vi "USB6343_Control_v1.6.5.vi"(8 "error in":errorcluster caption="错误输出", 10 "interface":T2, 11 "tasks":T3) -> ()   [LabVIEW 2013]
uses:
  <vilib>/DAQmx/read.llb/DAQmx Read (Analog 1D DBL NChan 1Samp).vi
  <vilib>/DAQmx/read.llb/DAQmx Read (Digital 1D Bool NChan 1Samp 1Line).vi
  <vilib>/DAQmx/read.llb/DAQmx Read (Counter DBL 1Chan 1Samp).vi
  <vilib>/DAQmx/write.llb/DAQmx Write (Digital 1D Bool NChan 1Samp 1Line).vi
  <vilib>/DAQmx/write.llb/DAQmx Write (Analog 1D DBL NChan 1Samp).vi
  current_position.vi
  <vilib>/DAQmx/miscellaneous.llb/DAQmx Fill In Error Info.vi
  <vilib>/DAQmx/configure/timing.llb/DAQmx Timing (Implicit).vi
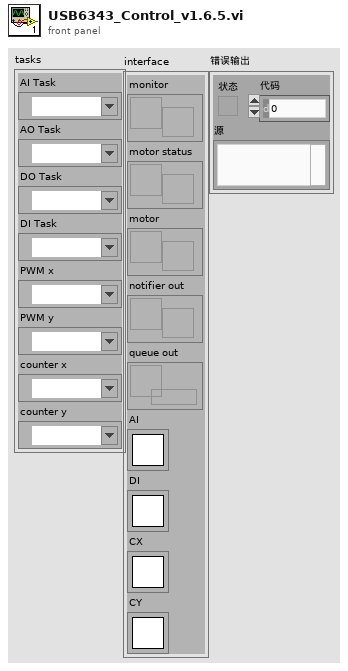
[diagram p1: front panel]
types:
  T1 = typedef "Semaphore RefNum" = refnum<k1>
  T2 = cluster{"monitor":refnum<user-event>, "motor status":refnum<user-event>, "motor":refnum<user-event>, "notifier out":refnum<notifier>, "queue out":refnum<queue>, "AI":T1, "DI":T1, "CX":T1, "CY":T1}
  T3 = cluster{"AI Task":refnum<k21>, "AO Task":refnum<k21>, "DO Task":refnum<k21>, "DI Task":refnum<k21>, "PWM x":refnum<k21>, "PWM y":refnum<k21>, "counter x":refnum<k21>, "counter y":refnum<k21>}
  T4 = cluster{"cmd":string, "channel":i32, "value":dbl, "on/off":bool, "return value":refnum<vi>}
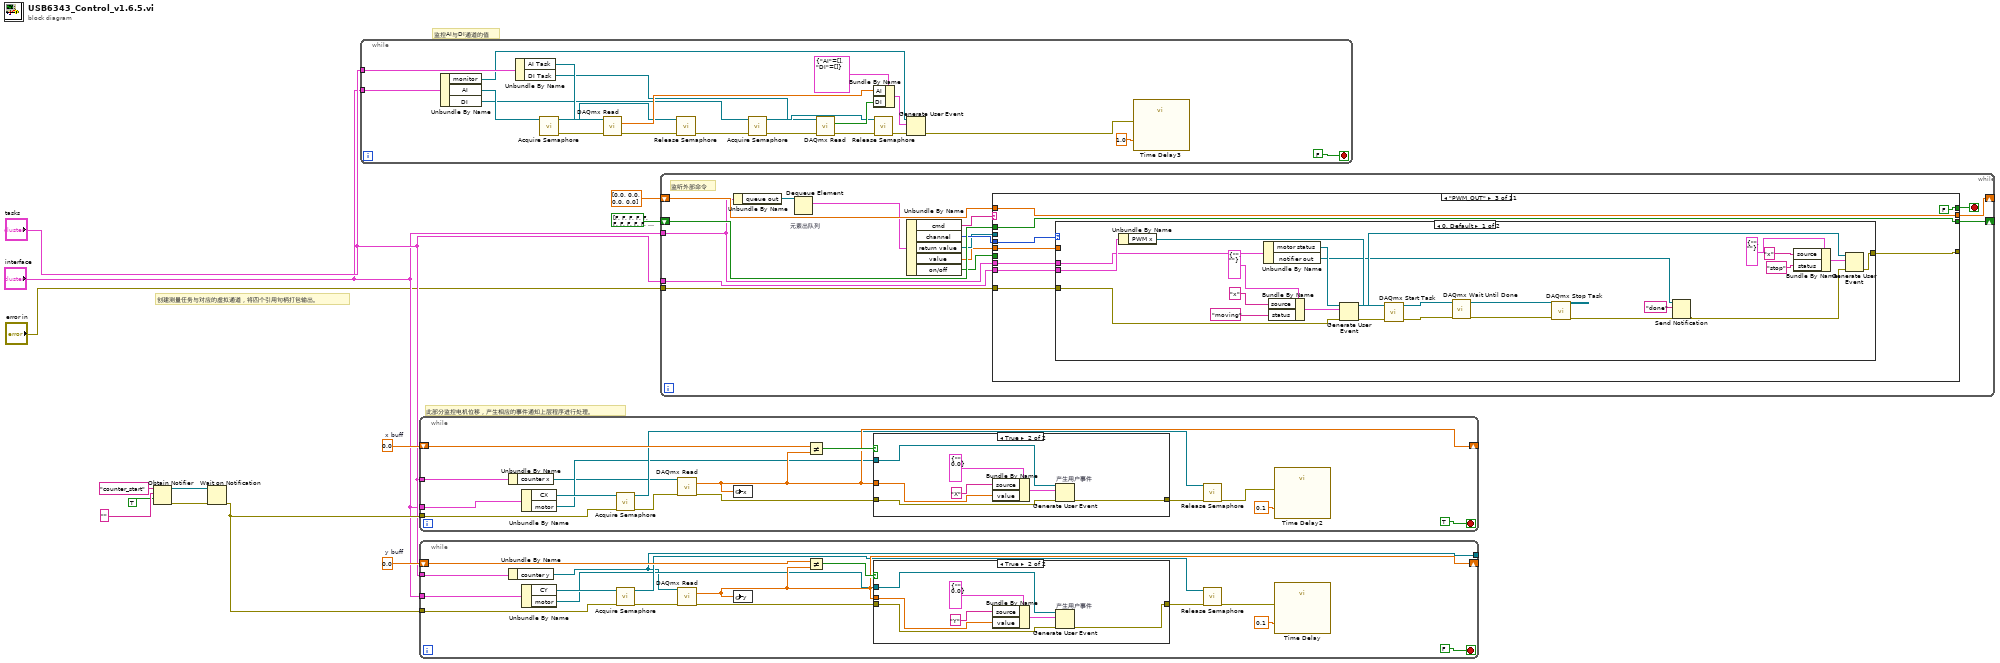
[diagram p0: block diagram]
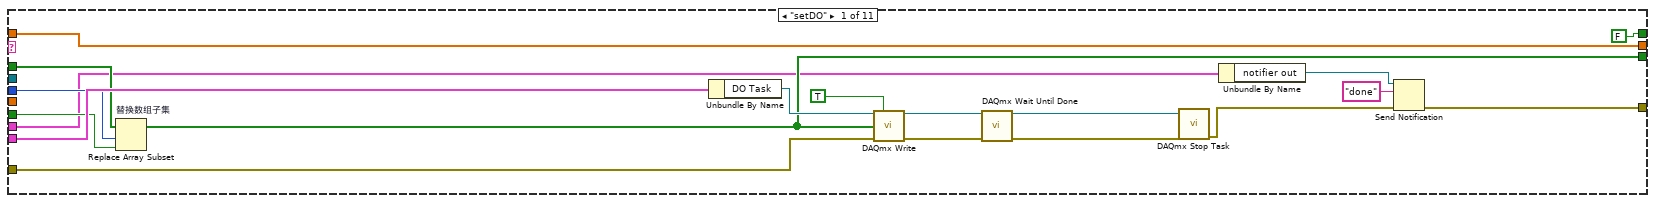
[diagram p4: hidden frame]
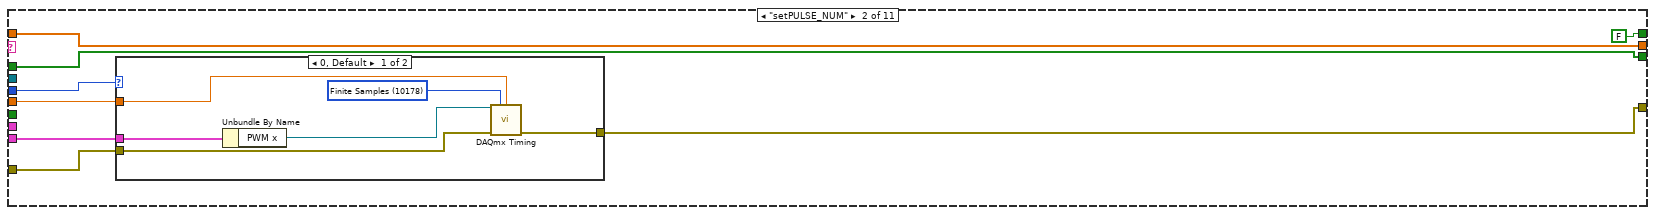
[diagram p5: hidden frame]
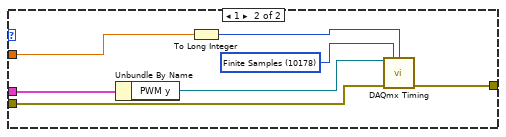
[diagram p6: hidden frame]
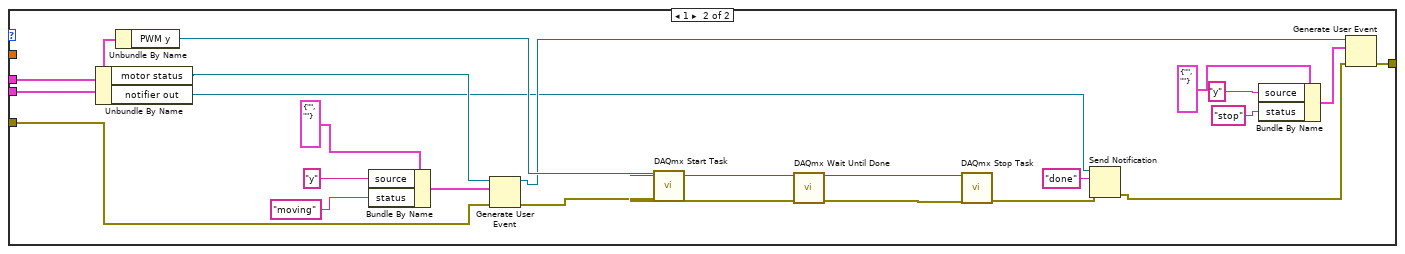
[diagram p7: hidden frame]
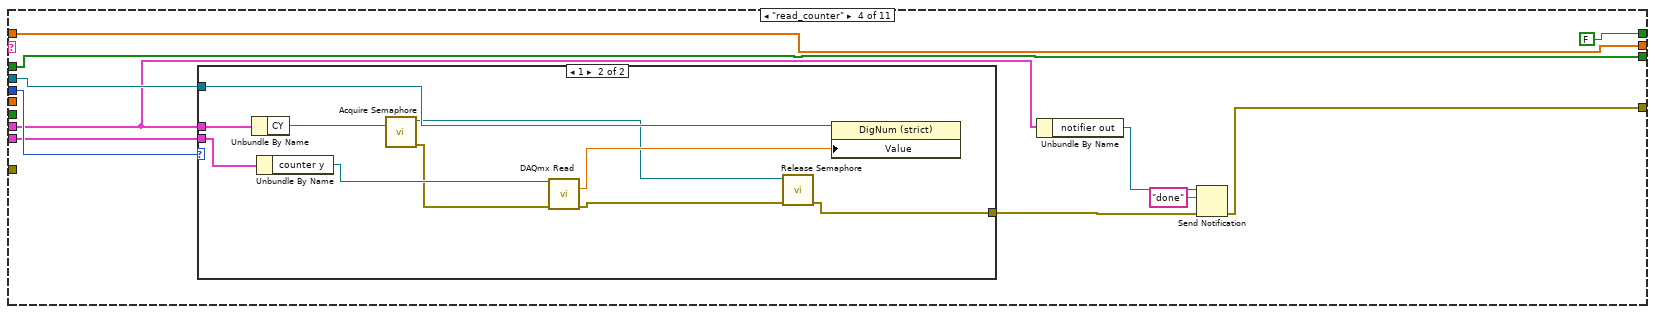
[diagram p8: hidden frame]
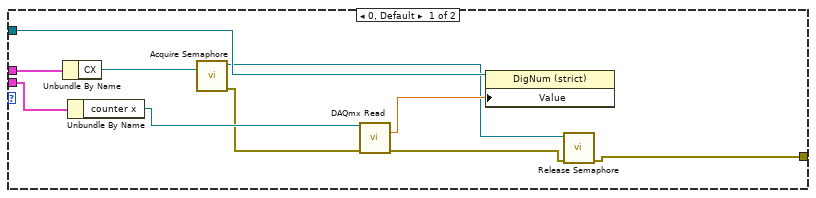
[diagram p9: hidden frame]
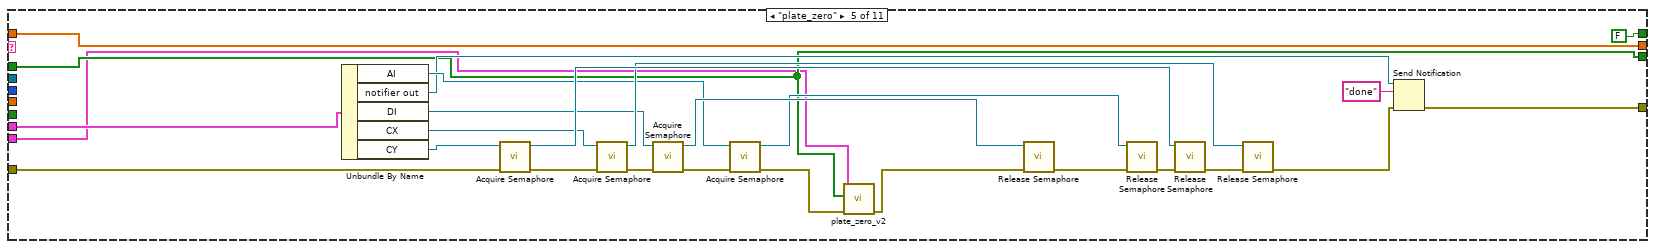
[diagram p10: hidden frame]
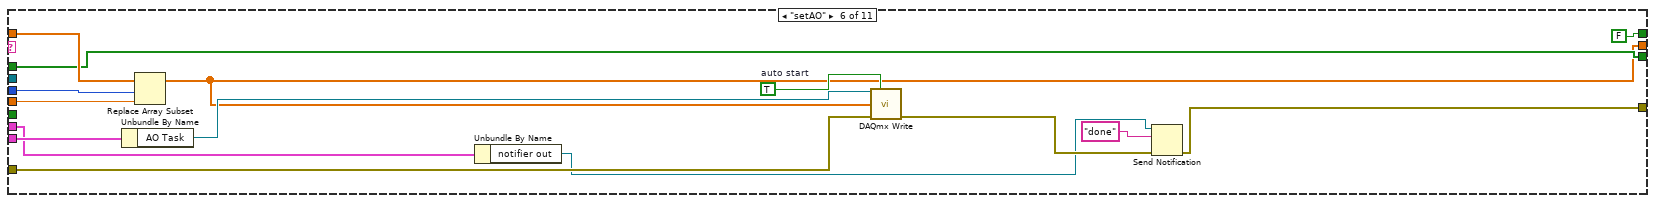
[diagram p11: hidden frame]
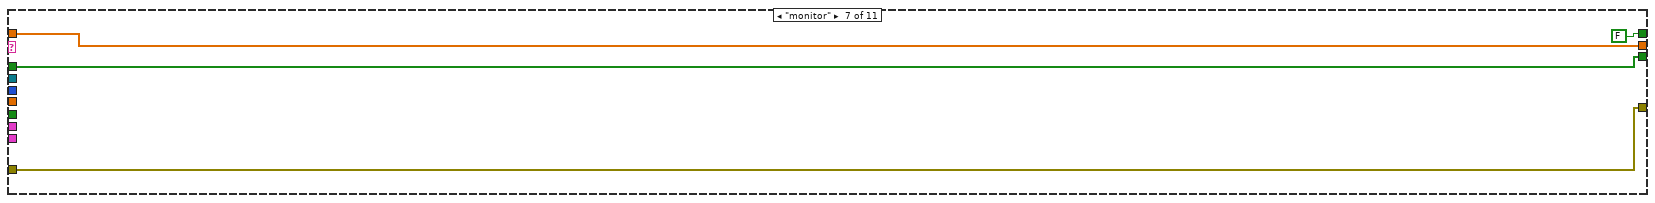
[diagram p12: hidden frame]
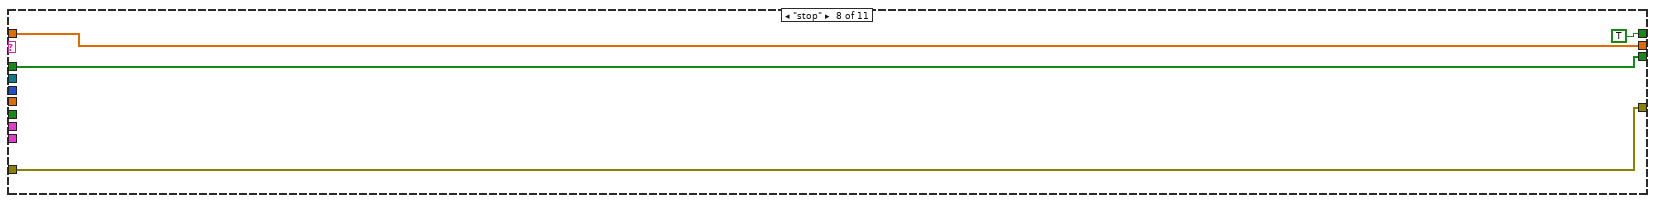
[diagram p13: hidden frame]
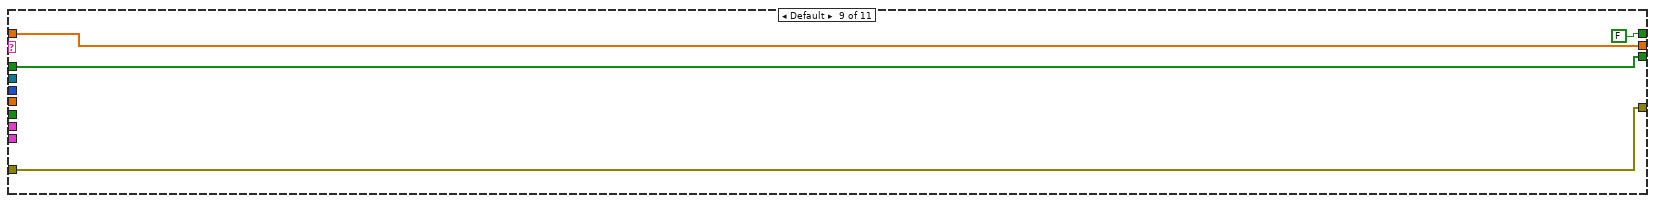
[diagram p14: hidden frame]
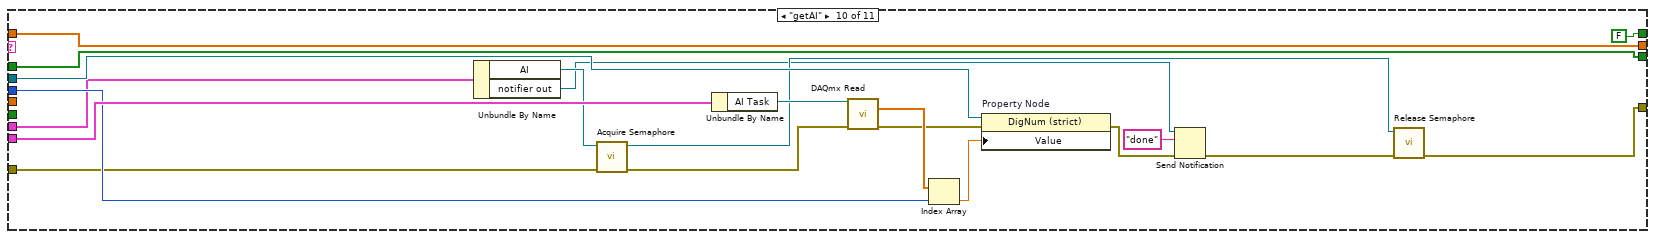
[diagram p15: hidden frame]
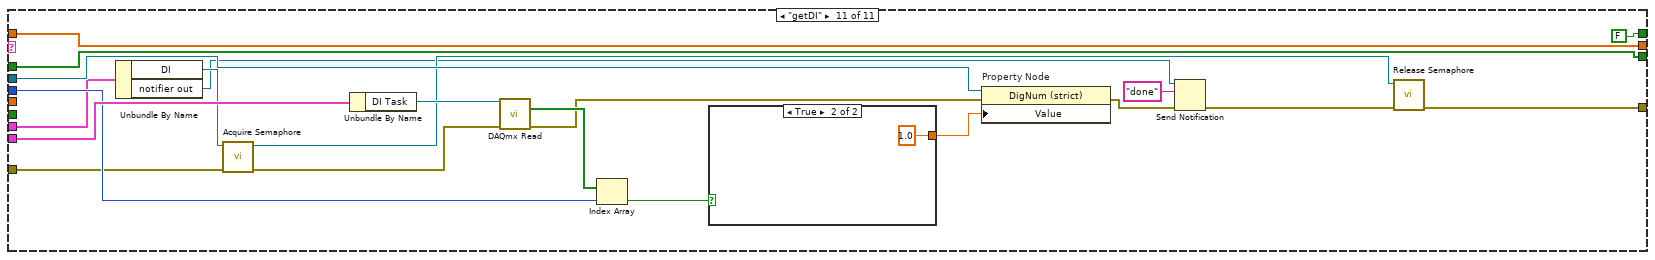
[diagram p16: hidden frame]
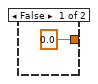
[diagram p17: hidden frame]
diagram:
  w10 = 0.0  # x buff
  w11 = 0.0  # y buff
  # "监控AI与DI通道的值"
  # "此部分监控电机位移，产生相应的事件通知上层程序进行处理。"
  # "创建测量任务与对应的虚拟通道，将四个引用句柄打包输出。"
  n1 = Obtain Notifier(name (unnamed)="counter_start", notification data type="", create if not found? (T)=TRUE) -> (notifier out=w6:refnum<notifier>, error out=w7:errorcluster)  [unwired: 1 in, 1 out]
  n2 = Wait on Notification(notifier=w6, error in (no error)=w7) -> (error out=w5:errorcluster)  [unwired: 2 in, 3 out]
  n3 = while {
    tunnel: "tasks" -> [w33]
    tunnel: "interface" -> [w18]
    stop <- FALSE stop-if-true
    n4 = Unbundle By Name(w18) -> ("monitor"=w17:refnum<user-event>, "AI"=w16:T1, "DI"=w15:T1)
    n5 = Unbundle By Name(w33) -> ("AI Task"=w34:refnum<k21>, "DI Task"=w14:refnum<k21>)
    n6 = call <vilib>:"Acquire Semaphore.vi"("semaphore"=w16) -> ("error out"=w19:errorcluster, "semaphore out"=w21:T1)  [unwired: 4 in, 1 out]
    n7 = call-poly <vilib>:"DAQmx Read.vi"("task/channels in"=w34, "error in"=w19) -> ("data"=w31:dbl[], "error out"=w26:errorcluster)  [unwired: 11 in, 1 out]
    n8 = call <vilib>:"Release Semaphore.vi"("error in (no error)"=w26, "semaphore"=w21) -> ("error out"=w25:errorcluster)  [unwired: 4 in, 1 out]
    n9 = call <vilib>:"Acquire Semaphore.vi"("error in (no error)"=w25, "semaphore"=w15) -> ("error out"=w24:errorcluster, "semaphore out"=w20:T1)  [unwired: 3 in, 1 out]
    n10 = call-poly <vilib>:"DAQmx Read.vi"("task/channels in"=w14, "error in"=w24) -> ("data"=w30:bool[], "error out"=w23:errorcluster)  [unwired: 11 in, 1 out]
    n11 = Bundle By Name(cluster=cluster{"AI":dbl[], "DI":bool[]} {"AI"=[], "DI"=[]} ("event data"), "AI"=w31, "DI"=w30) -> (w27:cluster{"AI":dbl[], "DI":bool[]})
    n12 = call <vilib>:"Release Semaphore.vi"("error in (no error)"=w23, "semaphore"=w20) -> ("error out"=w22:errorcluster)  [unwired: 4 in, 1 out]
    n13 = Generate User Event(user event=w17, event data cluster=w27, error in=w22) -> (error out=w29:errorcluster)  [unwired: 1 in, 1 out]
    n14 = call "Time Delay3"("error in (no error)"=w29, "Delay Time (s)"=1.0) -> ()  [unwired: 9 in, 1 out]
  }
  n15 = while {
    shift-right: [w47] -> _
    shift-left: w10 -> [w51]
    tunnel: "interface" -> [w41]
    tunnel: "tasks" -> [w38]
    tunnel: w5 -> [w36]
    stop <- TRUE stop-if-true
    n16 = Unbundle By Name(w38) -> ("counter x"=w37:refnum<k21>)
    n17 = Unbundle By Name(w41) -> ("CX"=w40:T1, "motor"=w39:refnum<user-event>)
    n18 = call <vilib>:"Acquire Semaphore.vi"("error in (no error)"=w36, "semaphore"=w40) -> ("error out"=w46:errorcluster, "semaphore out"=w43:T1)  [unwired: 3 in, 1 out]
    n19 = call-poly <vilib>:"DAQmx Read.vi"("task/channels in"=w37, "error in"=w46) -> ("data"=w47:dbl, "error out"=w49:errorcluster)  [unwired: 11 in, 1 out]
    n20 = global write "current_position.vi" "x"(w47) -> ()
    n21 = Not Equal?(x=w51, y=w47) -> (x != y?=w50:bool)
    n22 = case shown="True" w50 {
      tunnel: w47 -> [_ w53]
      tunnel: w49 -> [w52 w56]
      tunnel: [w52 w55] -> w45
      tunnel: w39 -> [_ w54]
      frame False {
      }
      frame True {
        n23 = Bundle By Name(cluster=cluster{"source":string, "value":dbl} {"source"="", "value"=0.0} ("事件数据"), "source"="X", "value"=w53) -> (w57:cluster{"source":string, "value":dbl})
        n24 = Generate User Event "产生用户事件"(user event=w54, event data cluster=w57, error in=w56) -> (error out=w55:errorcluster)  [unwired: 1 in, 1 out]
      }
    }
    n25 = call <vilib>:"Release Semaphore.vi"("error in (no error)"=w45, "semaphore"=w43) -> ("error out"=w44:errorcluster)  [unwired: 4 in, 1 out]
    n26 = call "Time Delay2"("error in (no error)"=w44, "Delay Time (s)"=0.1) -> ()  [unwired: 9 in, 1 out]
  }
  n27 = while {
    tunnel: [w61] -> _
    shift-right: [w71] -> _
    shift-left: w11 -> [w75]
    tunnel: "interface" -> [w65]
    tunnel: "tasks" -> [w62]
    tunnel: w5 -> [w60]
    stop <- FALSE stop-if-true
    n28 = Unbundle By Name(w62) -> ("counter y"=w61:refnum<k21>)
    n29 = Unbundle By Name(w65) -> ("CY"=w64:T1, "motor"=w63:refnum<user-event>)
    n30 = call <vilib>:"Acquire Semaphore.vi"("error in (no error)"=w60, "semaphore"=w64) -> ("error out"=w70:errorcluster, "semaphore out"=w67:T1)  [unwired: 3 in, 1 out]
    n31 = call-poly <vilib>:"DAQmx Read.vi"("task/channels in"=w61, "error in"=w70) -> ("data"=w71:dbl, "error out"=w73:errorcluster)  [unwired: 11 in, 1 out]
    n32 = global write "current_position.vi" "y"(w71) -> ()
    n33 = Not Equal?(x=w75, y=w71) -> (x != y?=w74:bool)
    n34 = case shown="True" w74 {
      tunnel: w71 -> [_ w77]
      tunnel: w73 -> [w76 w79]
      tunnel: [w76 w78] -> w69
      tunnel: w63 -> [_ w80]
      frame False {
      }
      frame True {
        n35 = Bundle By Name(cluster=cluster{"source":string, "value":dbl} {"source"="", "value"=0.0} ("事件数据"), "source"="Y", "value"=w77) -> (w81:cluster{"source":string, "value":dbl})
        n36 = Generate User Event "产生用户事件"(user event=w80, event data cluster=w81, error in=w79) -> (error out=w78:errorcluster)  [unwired: 1 in, 1 out]
      }
    }
    n37 = call <vilib>:"Release Semaphore.vi"("error in (no error)"=w69, "semaphore"=w67) -> ("error out"=w68:errorcluster)  [unwired: 4 in, 1 out]
    n38 = call "Time Delay"("error in (no error)"=w68, "Delay Time (s)"=0.1) -> ()  [unwired: 9 in, 1 out]
  }
  n39 = while {
    tunnel: "tasks" -> [w92]
    tunnel: "error in" -> [w98]
    shift-right: [w96] -> _
    shift-left: bool[] [FALSE, FALSE, FALSE, FALSE, FALSE, FALSE, FALSE, FALSE, FALSE, FALSE, FALSE, FALSE, FALSE, FALSE, FALSE, FALSE] -> [w97]
    shift-right: [w93] -> _
    shift-left: dbl[] [0.0, 0.0, 0.0, 0.0] ("data") -> [w94]
    tunnel: "interface" -> [w85]
    stop <- w95 stop-if-true
    # "监听外部命令"
    n40 = Unbundle By Name(w85) -> ("queue out"=w84:refnum<queue>)
    n41 = Dequeue Element "元素出队列"(queue=w84) -> (element=w91:T4)  [unwired: 2 in, 3 out]
    n42 = Unbundle By Name(w91) -> ("cmd"=w90:string, "channel"=w89:i32, "return value"=w88:refnum<vi>, "value"=w86:dbl, "on/off"=w87:bool)
    n43 = case shown="\"PWM_OUT\"" w90 {
      tunnel: w89 -> [w115 w119 w141 w206 _ w265 _ _ _ w295 w318]
      tunnel: w92 -> [w117 w122 w144 w205 w228 w267 _ _ _ w299 w320]
      tunnel: w98 -> [w109 w120 w142 _ w244 w260 w268 w272 w276 w288 w308]
      tunnel: w97 -> [w116 w123 w145 w196 w230 w263 w271 w275 w279 w293 w317]
      tunnel: w87 -> [w114 _ _ _ _ _ _ _ _ _ _]
      tunnel: [w107 w123 w145 w196 w230 w263 w271 w275 w279 w293 w317] -> w96
      tunnel: [FALSE FALSE FALSE FALSE FALSE FALSE FALSE TRUE FALSE FALSE FALSE] -> w95
      tunnel: w94 -> [w112 w124 w146 w197 w251 w264 w270 w273 w277 w292 w316]
      tunnel: [w112 w124 w146 w197 w251 w253 w270 w273 w277 w292 w316] -> w93
      tunnel: w88 -> [_ _ _ w204 _ _ _ _ _ w297 w319]
      tunnel: [w111 w118 w140 w199 w250 w257 w268 w272 w276 w284 w303] -> _
      tunnel: w86 -> [_ w121 w143 _ _ w259 _ _ _ _ _]
      tunnel: w85 -> [w103 _ w139 w202 w236 w256 _ _ _ w282 w302]
      frame "setDO" {
        n44 = Replace Array Subset "替换数组子集"(array=w116, new element=w114, index=w115) -> (w107:bool[])
        n45 = Unbundle By Name(w117) -> ("DO Task"=w108:refnum<k21>)
        n46 = call-poly <vilib>:"DAQmx Write.vi"("task/channels in"=w108, "auto start"=TRUE, "data"=w107, "error in"=w109) -> ("task out"=w104:refnum<k21>, "error out"=w105:errorcluster)  [unwired: 9 in, 1 out]
        n47 = call <vilib>:"DAQmx Wait Until Done.vi"("task/channels in"=w104, "error in"=w105) -> ("task out"=w99:refnum<k21>, "error out"=w101:errorcluster)  [unwired: 12 in]
        n48 = call <vilib>:"DAQmx Stop Task.vi"("task/channels in"=w99, "error in"=w101) -> ("error out"=w100:errorcluster)  [unwired: 12 in, 1 out]
        n49 = Unbundle By Name(w103) -> ("notifier out"=w102:refnum<notifier>)
        n50 = Send Notification(notification="done" ("通知"), notifier=w102, error in (no error)=w100) -> (error out=w111:errorcluster)  [unwired: 1 out]
      }
      frame "setPULSE_NUM" {
        n51 = case shown="0, Default" w119 {
          tunnel: w122 -> [w131 w138]
          tunnel: w121 -> [w128 w133]
          tunnel: w120 -> [w127 w135]
          tunnel: [w126 w134] -> w118
          frame 0, Default {
            w129 = 10178 items=["Finite Samples"=10178, "Continuous Samples"=10123, "Hardware Timed Single Point"=12522] ("sample mode")
            n52 = Unbundle By Name(w131) -> ("PWM x"=w130:refnum<k21>)
            n53 = call-poly <vilib>:"DAQmx Timing.vi"("task/channels in"=w130, "sample mode"=w129, "samples per channel"=w128, "error in"=w127) -> ("error out"=w126:errorcluster)  [unwired: 10 in, 1 out]
          }
          frame 1 {
            w136 = 10178 items=["Finite Samples"=10178, "Continuous Samples"=10123, "Hardware Timed Single Point"=12522] ("sample mode")
            n54 = Unbundle By Name(w138) -> ("PWM y"=w137:refnum<k21>)
            n55 = To Long Integer(number=w133) -> (32bit integer=w132:i32)
            n56 = call-poly <vilib>:"DAQmx Timing.vi"("task/channels in"=w137, "sample mode"=w136, "samples per channel"=w132, "error in"=w135) -> ("error out"=w134:errorcluster)  [unwired: 10 in, 1 out]
          }
        }
      }
      frame "PWM_OUT" {
        n57 = case shown="0, Default" w141 {
          tunnel: w144 -> [w171 w195]
          tunnel: w143 -> [_ _]
          tunnel: w142 -> [w163 w187]
          tunnel: [w156 w181] -> w140
          tunnel: w139 -> [w154 w178]
          frame 0, Default {
            n58 = Unbundle By Name(w171) -> ("PWM x"=w170:refnum<k21>)
            n59 = Unbundle By Name(w154) -> ("motor status"=w153:refnum<user-event>, "notifier out"=w148:refnum<notifier>)
            n60 = Bundle By Name(cluster=cluster{"source":string, " status":string} {"source"="", " status"=""} ("event data"), "source"="x", "status"="moving") -> (w161:cluster{"source":string, " status":string})
            n61 = Generate User Event(user event=w153, event data cluster=w161, error in=w163) -> (user event out=w155:refnum<user-event>, error out=w162:errorcluster)  [unwired: 1 in]
            n62 = call <vilib>:"DAQmx Start Task.vi"("task/channels in"=w170, "error in"=w162) -> ("task out"=w168:refnum<k21>, "error out"=w169:errorcluster)  [unwired: 12 in]
            n63 = call <vilib>:"DAQmx Wait Until Done.vi"("task/channels in"=w168, "error in"=w169) -> ("task out"=w167:refnum<k21>, "error out"=w152:errorcluster)  [unwired: 12 in]
            n64 = call <vilib>:"DAQmx Stop Task.vi"("task/channels in"=w167, "error in"=w152) -> ("error out"=w151:errorcluster)  [unwired: 12 in, 1 out]
            n65 = Send Notification(notification="done", notifier=w148, error in (no error)=w151) -> (error out=w150:errorcluster)  [unwired: 1 out]
            n66 = Bundle By Name(cluster=cluster{"source":string, " status":string} {"source"="", " status"=""} ("event data"), "source"="x", "status"="stop") -> (w157:cluster{"source":string, " status":string})
            n67 = Generate User Event(user event=w155, event data cluster=w157, error in=w150) -> (error out=w156:errorcluster)  [unwired: 1 in, 1 out]
          }
          frame 1 {
            n68 = Unbundle By Name(w178) -> ("motor status"=w177:refnum<user-event>, "notifier out"=w172:refnum<notifier>)
            n69 = Unbundle By Name(w195) -> ("PWM y"=w194:refnum<k21>)
            n70 = Bundle By Name(cluster=cluster{"source":string, " status":string} {"source"="", " status"=""} ("event data"), "source"="y", "status"="moving") -> (w180:cluster{"source":string, " status":string})
            n71 = Generate User Event(user event=w177, event data cluster=w180, error in=w187) -> (user event out=w176:refnum<user-event>, error out=w186:errorcluster)  [unwired: 1 in]
            n72 = call <vilib>:"DAQmx Start Task.vi"("task/channels in"=w194, "error in"=w186) -> ("task out"=w192:refnum<k21>, "error out"=w193:errorcluster)  [unwired: 12 in]
            n73 = call <vilib>:"DAQmx Wait Until Done.vi"("task/channels in"=w192, "error in"=w193) -> ("task out"=w190:refnum<k21>, "error out"=w191:errorcluster)  [unwired: 12 in]
            n74 = call <vilib>:"DAQmx Stop Task.vi"("task/channels in"=w190, "error in"=w191) -> ("error out"=w175:errorcluster)  [unwired: 12 in, 1 out]
            n75 = Send Notification(notification="done", notifier=w172, error in (no error)=w175) -> (error out=w174:errorcluster)  [unwired: 1 out]
            n76 = Bundle By Name(cluster=cluster{"source":string, " status":string} {"source"="", " status"=""} ("event data"), "source"="y", "status"="stop") -> (w182:cluster{"source":string, " status":string})
            n77 = Generate User Event(user event=w176, event data cluster=w182, error in=w174) -> (error out=w181:errorcluster)  [unwired: 1 in, 1 out]
          }
        }
      }
      frame "read_counter" {
        n78 = case shown="1" w206 {
          tunnel: w202 -> [w216 w226]
          tunnel: w205 -> [w214 w224]
          tunnel: w204 -> [w211 w221]
          tunnel: [w207 w217] -> w203
          frame 0, Default {
            n79 = Unbundle By Name(w216) -> ("CX"=w215:T1)
            n80 = Unbundle By Name(w214) -> ("counter x"=w213:refnum<k21>)
            n81 = call <vilib>:"Acquire Semaphore.vi"("semaphore"=w215) -> ("error out"=w212:errorcluster, "semaphore out"=w208:T1)  [unwired: 4 in, 1 out]
            n82 = call-poly <vilib>:"DAQmx Read.vi"("task/channels in"=w213, "error in"=w212) -> ("data"=w210:dbl, "error out"=w209:errorcluster)  [unwired: 11 in, 1 out]
            n83 = property class="DigNum (strict)"(reference=w211, "Value"=w210) -> ()  [unwired: 1 in, 2 out]
            n84 = call <vilib>:"Release Semaphore.vi"("error in (no error)"=w209, "semaphore"=w208) -> ("error out"=w207:errorcluster)  [unwired: 4 in, 1 out]
          }
          frame 1 {
            n85 = Unbundle By Name(w226) -> ("CY"=w225:T1)
            n86 = Unbundle By Name(w224) -> ("counter y"=w223:refnum<k21>)
            n87 = call <vilib>:"Acquire Semaphore.vi"("semaphore"=w225) -> ("error out"=w222:errorcluster, "semaphore out"=w218:T1)  [unwired: 4 in, 1 out]
            n88 = call-poly <vilib>:"DAQmx Read.vi"("task/channels in"=w223, "error in"=w222) -> ("data"=w220:dbl, "error out"=w219:errorcluster)  [unwired: 11 in, 1 out]
            n89 = call <vilib>:"Release Semaphore.vi"("error in (no error)"=w219, "semaphore"=w218) -> ("error out"=w217:errorcluster)  [unwired: 4 in, 1 out]
            n90 = property class="DigNum (strict)"(reference=w221, "Value"=w220) -> ()  [unwired: 1 in, 2 out]
          }
        }
        n91 = Unbundle By Name(w202) -> ("notifier out"=w201:refnum<notifier>)
        n92 = Send Notification(notification="done", notifier=w201, error in (no error)=w203) -> (error out=w199:errorcluster)  [unwired: 1 out]
      }
      frame "plate_zero" {
        n93 = Unbundle By Name(w236) -> ("AI"=w235:T1, "notifier out"=w231:refnum<notifier>, "DI"=w234:T1, "CX"=w233:T1, "CY"=w232:T1)
        n94 = call <vilib>:"Acquire Semaphore.vi"("error in (no error)"=w244, "semaphore"=w232) -> ("error out"=w246:errorcluster, "semaphore out"=w240:T1)  [unwired: 3 in, 1 out]
        n95 = call <vilib>:"Acquire Semaphore.vi"("error in (no error)"=w246, "semaphore"=w233) -> ("error out"=w245:errorcluster, "semaphore out"=w237:T1)  [unwired: 3 in, 1 out]
        n96 = call <vilib>:"Acquire Semaphore.vi"("error in (no error)"=w245, "semaphore"=w234) -> ("error out"=w248:errorcluster, "semaphore out"=w239:T1)  [unwired: 3 in, 1 out]
        n97 = call <vilib>:"Acquire Semaphore.vi"("error in (no error)"=w248, "semaphore"=w235) -> ("error out"=w229:errorcluster, "semaphore out"=w238:T1)  [unwired: 3 in, 1 out]
        n98 = call "plate_zero_v2.vi"("error in"=w229, "DO array"=w230, "tasks"=w228) -> ("error out"=w227:errorcluster)  [unwired: 8 in]
        n99 = call <vilib>:"Release Semaphore.vi"("error in (no error)"=w227, "semaphore"=w239) -> ("error out"=w247:errorcluster)  [unwired: 4 in, 1 out]
        n100 = call <vilib>:"Release Semaphore.vi"("error in (no error)"=w247, "semaphore"=w238) -> ("error out"=w243:errorcluster)  [unwired: 4 in, 1 out]
        n101 = call <vilib>:"Release Semaphore.vi"("error in (no error)"=w243, "semaphore"=w240) -> ("error out"=w242:errorcluster)  [unwired: 4 in, 1 out]
        n102 = call <vilib>:"Release Semaphore.vi"("error in (no error)"=w242, "semaphore"=w237) -> ("error out"=w241:errorcluster)  [unwired: 4 in, 1 out]
        n103 = Send Notification(notification="done", notifier=w231, error in (no error)=w241) -> (error out=w250:errorcluster)  [unwired: 1 out]
      }
      frame "setAO" {
        w262 = TRUE  # auto start
        n104 = Unbundle By Name(w267) -> ("AO Task"=w266:refnum<k21>)
        n105 = Replace Array Subset(array=w264, new element=w259, index=w265) -> (w253:dbl[])
        n106 = Unbundle By Name(w256) -> ("notifier out"=w255:refnum<notifier>)
        n107 = call-poly <vilib>:"DAQmx Write.vi"("task/channels in"=w266, "auto start"=w262, "data"=w253, "error in"=w260) -> ("error out"=w258:errorcluster)  [unwired: 9 in, 2 out]
        n108 = Send Notification(notification="done", notifier=w255, error in (no error)=w258) -> (error out=w257:errorcluster)  [unwired: 1 out]
      }
      frame "monitor" {
      }
      frame "stop" {
      }
      frame Default {
      }
      frame "getAI" {
        n109 = Unbundle By Name(w282) -> ("AI"=w281:T1, "notifier out"=w280:refnum<notifier>)
        n110 = call <vilib>:"Acquire Semaphore.vi"("error in (no error)"=w288, "semaphore"=w281) -> ("error out"=w287:errorcluster, "semaphore out"=w283:T1)  [unwired: 3 in, 1 out]
        n111 = Unbundle By Name(w299) -> ("AI Task"=w298:refnum<k21>)
        n112 = call-poly <vilib>:"DAQmx Read.vi"("task/channels in"=w298, "error in"=w287) -> ("data"=w296:dbl[], "error out"=w286:errorcluster)  [unwired: 11 in, 1 out]
        n113 = Index Array(array=w296, index=w295) -> (element=w294:dbl)
        n114 = property on="Property Node" class="DigNum (strict)"(reference=w297, error in=w286, "Value"=w294) -> (error out=w289:errorcluster)  [unwired: 1 out]
        n115 = Send Notification(notification="done" ("通知"), notifier=w280, error in (no error)=w289) -> (error out=w285:errorcluster)  [unwired: 1 out]
        n116 = call <vilib>:"Release Semaphore.vi"("error in (no error)"=w285, "semaphore"=w283) -> ("error out"=w284:errorcluster)  [unwired: 4 in, 1 out]
      }
      frame "getDI" {
        n117 = Unbundle By Name(w302) -> ("DI"=w301:T1, "notifier out"=w300:refnum<notifier>)
        n118 = call <vilib>:"Acquire Semaphore.vi"("error in (no error)"=w308, "semaphore"=w301) -> ("error out"=w307:errorcluster, "semaphore out"=w304:T1)  [unwired: 3 in, 1 out]
        n119 = Unbundle By Name(w320) -> ("DI Task"=w312:refnum<k21>)
        n120 = call-poly <vilib>:"DAQmx Read.vi"("task/channels in"=w312, "error in"=w307) -> ("data"=w311:bool[], "error out"=w306:errorcluster)  [unwired: 11 in, 1 out]
        n121 = Index Array "Index Array"(array=w311, index=w318) -> (element=w310:bool)
        n122 = case shown="True" w310 {
          tunnel: [0.0 1.0] -> w309
          frame False {
          }
          frame True {
          }
        }
        n123 = property on="Property Node" class="DigNum (strict)"(reference=w319, error in=w306, "Value"=w309) -> (error out=w313:errorcluster)  [unwired: 1 out]
        n124 = Send Notification(notification="done" ("通知"), notifier=w300, error in (no error)=w313) -> (error out=w305:errorcluster)  [unwired: 1 out]
        n125 = call <vilib>:"Release Semaphore.vi"("error in (no error)"=w305, "semaphore"=w304) -> ("error out"=w303:errorcluster)  [unwired: 4 in, 1 out]
      }
    }
  }
